vi "AnalyseBands.vi"(10 "SearchBands":cluster{"Min":dbl, "Max":dbl, "Name":string}[](array[cluster])=[{"Min"=40.0, "Max"=70.0, "Name"=""}, {"Min"=100.0, "Max"=140.0, "Name"=""}, {"Min"=450.0, "Max"=510.0, "Name"=""}, {"Min"=600.0, "Max"=680.0, "Name"=""}]) -> (2 "Results":string[][](array[string]))   [LabVIEW 2014]
uses:
  Globals/Meas_global.vi
panel:
  in  "MicsToAnalyse":bool[](array[boolean])=[TRUE, FALSE, FALSE, FALSE]
  in  "GraphDisplay":bool
  out "XY Graph":T1(graph)
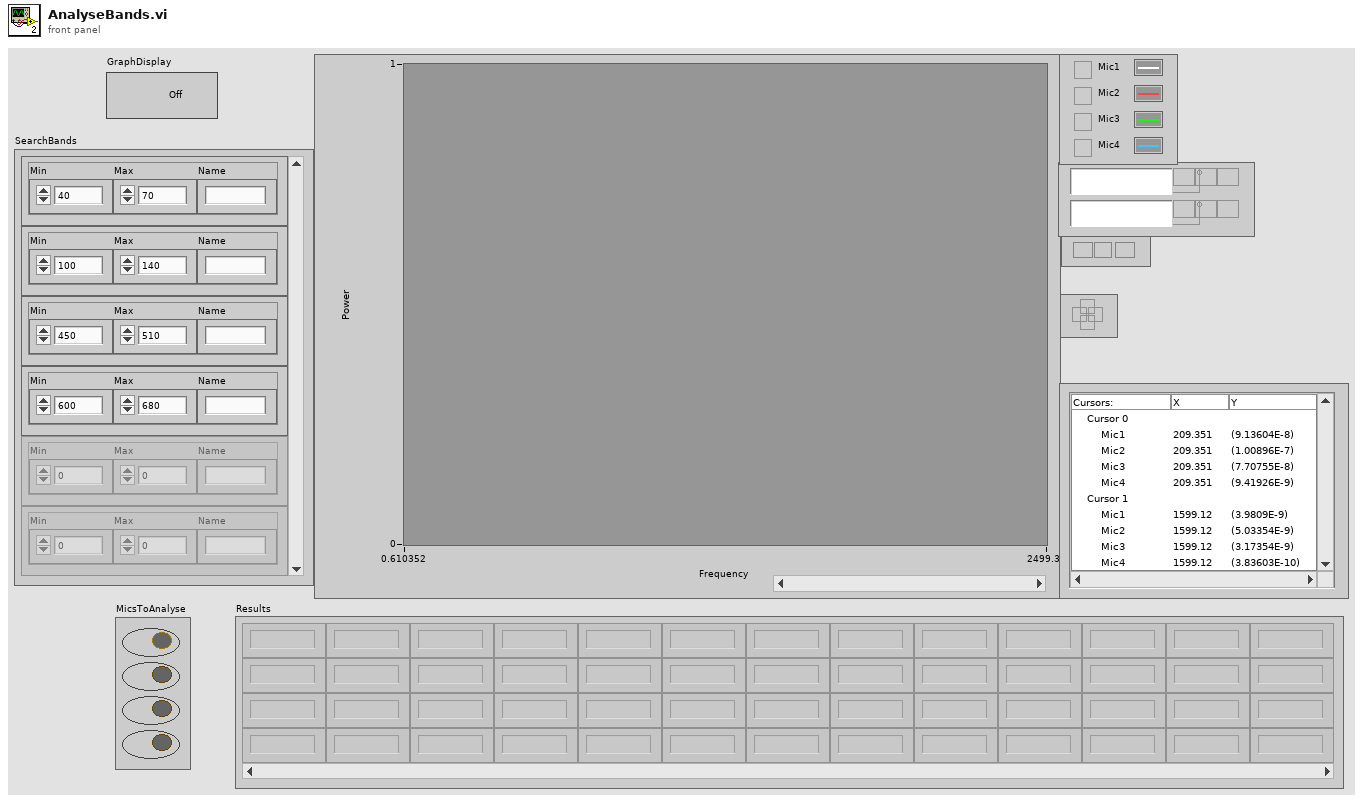
[diagram p1: front panel]
types:
  T1 = cluster{"Frequencies":dbl[], "Spectrum output array":dbl[]}[]
  T2 = typedef "Time_Trace_Cluster.ctl" = cluster{"Weighting":dbl[], "Time (s)":dbl[], "Voltage":dbl[], "Eng Values":dbl[]}
  T3 = cluster{"Frequencies":dbl[], "Spectrum output array":dbl[]}
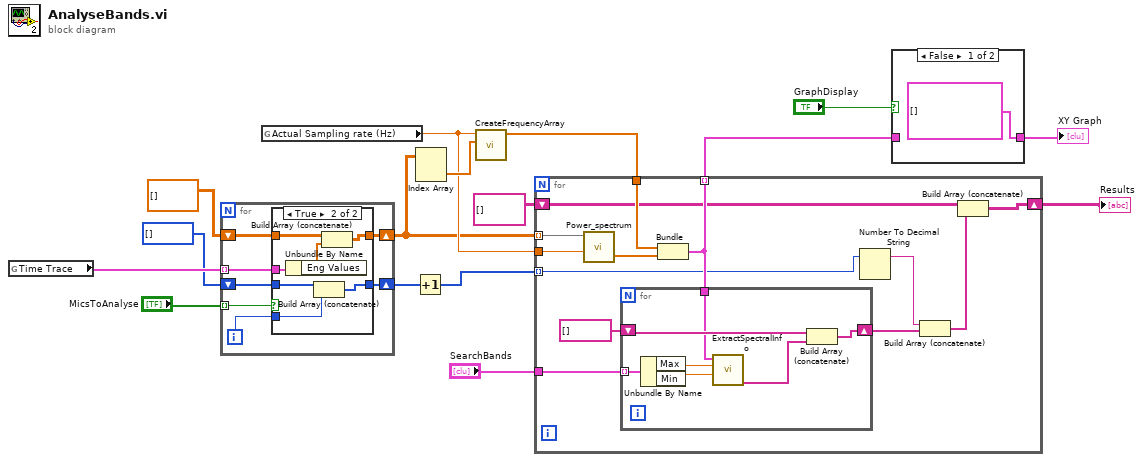
[diagram p0: block diagram]
diagram:
  n1 = global read "Meas_global.vi" "Time Trace"() -> (w7:T2[])
  n2 = for {
    tunnel: w7 -> [w23] mode=indexing
    shift-right: [w21] -> w6
    shift-left: dbl[][] [] -> [w22]
    shift-right: [w20] -> w5
    shift-left: i32[] [] -> [w19]
    tunnel: "MicsToAnalyse" -> [w18] mode=indexing
    i -> [w17]
    n3 = case shown="True" w18 {
      tunnel: w23 -> [_ w32]
      tunnel: w22 -> [w25 w30]
      tunnel: [w25 w29] -> w21
      tunnel: [w24 w27] -> w20
      tunnel: w19 -> [w24 w28]
      tunnel: w17 -> [_ w26]
      frame False {
      }
      frame True {
        n4 = Unbundle By Name(w32) -> ("Eng Values"=w31:dbl[])
        n5 = Build Array (concatenate)(w28, w26) -> (w27:i32[])
        n6 = Build Array (concatenate)(w30, w31) -> (w29:dbl[][])
      }
    }
  }
  n7 = global read "Meas_global.vi" "Actual Sampling rate (Hz)"() -> (w12:dbl)
  n8 = Increment(x=w5) -> (x+1=w2:i32[])
  n9 = Index Array(array=w6) -> (element=w16:dbl[])  [unwired: 2 in]
  n10 = call "CreateFrequencyArray.vi"("Signal"=w16, "Actual Sampling rate (Hz)"=w12) -> ("Frequencies"=w15:dbl[])  [unwired: 9 in]
  n11 = for {
    tunnel: w12 -> [w45]
    tunnel: [w44] -> w13 mode=indexing
    tunnel: w15 -> [w43]
    tunnel: w6 -> [w41] mode=indexing
    shift-right: [w40] -> w8
    shift-left: string[][] [] -> [w38]
    tunnel: "SearchBands" -> [w39]
    tunnel: w2 -> [w33] mode=indexing
    n12 = call "Power_spectrum.vi"("U"=w41, "Sampling frequency"=w45) -> ("Spectrum output array"=w42:dbl[])  [unwired: 3 in, 1 out]
    n13 = Bundle("Frequencies"=w43, "Spectrum output array"=w42) -> (w44:T3)  [unwired: 1 out]
    n14 = for {
      tunnel: w44 -> [w47]
      tunnel: w39 -> [w50] mode=indexing
      shift-right: [w49] -> w37
      shift-left: string[] [] -> [w48]
      n15 = Unbundle By Name(w50) -> ("Max"=w52:dbl, "Min"=w51:dbl)
      n16 = call "ExtractSpectralInfo.vi"("Min"=w51, "Max"=w52, "Spectrum"=w47) -> ("Analysis"=w46:string[])  [unwired: 5 in, 3 out]
      n17 = Build Array (concatenate)(w48, w46) -> (w49:string[])
    }
    n18 = Number To Decimal String(number=w33) -> (decimal integer string=w34:string)  [unwired: 1 in]
    n19 = Build Array (concatenate)(w34, w37) -> (w36:string[])
    n20 = Build Array (concatenate)(w38, w36) -> (w40:string[][])
  }
  "Results" <- w8
  n21 = case shown="False" "GraphDisplay" {
    tunnel: w13 -> [_ w54]
    tunnel: [T1 [] w54] -> w11
    frame False {
    }
    frame True {
    }
  }
  "XY Graph" <- w11
